vi "libmodbus Demo.vi"() -> ()   [LabVIEW 2017, in "libmodbus.lvlib"]
uses:
  libmodbus.lvlib
  libmodbus.lvclass
panel:
  in  "registers":u16[](array[numeric])=[1, 3]
  out "registers read":u16[](array[numeric])
  out "error out":errorcluster
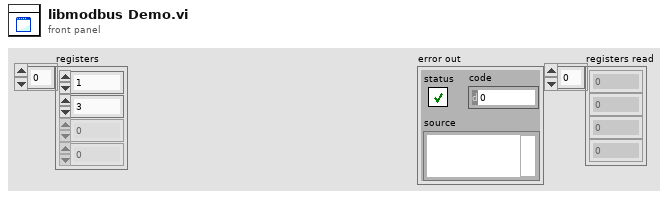
[diagram p1: front panel]
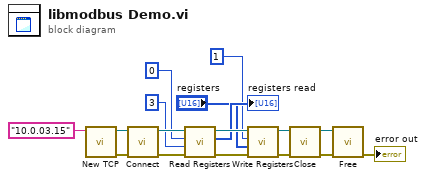
[diagram p0: block diagram]
diagram:
  n1 = call "New TCP.vi"("ip address"="10.0.03.15") -> ("error out"=w15:errorcluster, "modbus out"=w16:refnum<class "libmodbus.lvclass">)  [unwired: 9 in]
  n2 = call "Connect.vi"("error in (no error)"=w15, "modbus in"=w16) -> ("error out"=w9:errorcluster, "modbus out"=w11:refnum<class "libmodbus.lvclass">)  [unwired: 8 in]
  n3 = call "Read Registers.vi"("error in (no error)"=w9, "number of registers"=3, "address"=0, "modbus in"=w11) -> ("error out"=w3:errorcluster, "registers read"=→"registers read":u16[], "modbus out"=w10:refnum<class "libmodbus.lvclass">)  [unwired: 5 in]
  n4 = call "Write Registers.vi"("error in (no error)"=w3, "registers"="registers", "address"=1, "modbus in"=w10) -> ("error out"=w2:errorcluster, "modbus out"=w1:refnum<class "libmodbus.lvclass">)  [unwired: 6 in]
  n5 = call "Close.vi"("error in (no error)"=w2, "modbus in"=w1) -> ("error out"=w13:errorcluster, "modbus out"=w12:refnum<class "libmodbus.lvclass">)  [unwired: 8 in]
  n6 = call "Free.vi"("error in (no error)"=w13, "modbus in"=w12) -> ("error out"=→"error out":errorcluster)  [unwired: 9 in]
